vi "Create IRegisteredHandler.vi"(8 "error in (no error)":errorcluster, 11 "IWampMessage":refnum<class "IWampMessage.lvclass">) -> (0 "error out":errorcluster, 3 "IRegisteredHandler out":refnum<class "IRegisteredHandler.lvclass">)   [LabVIEW 2020, in "wamplv.lvlib"]
uses:
  wamplv.lvlib
  IRegisteredHandler.lvclass
  SerialisedMessages/IWampMessage/IWampMessage.lvclass
  RegisteredHandler JSON/RegisteredHandler JSON.lvclass
  C:/local/wamplv/Private/Requests/MessageReceivedHandlers/Registered/IRegisteredHandler.lvclass
  C:/local/wamplv/Private/Requests/MessageReceivedHandlers/IJsonMessageHandler/IJsonMessageHandler.lvclass
  SerialisedMessages/JSONMessage/JSONMessage.lvclass
  IJsonMessageHandler/IJsonMessageHandler.lvclass/IJsonMessageHandler.ctl
  RegisteredHandler MsgPack/RegisteredHandler MsgPack.lvclass
  C:/local/wamplv/Private/Requests/MessageReceivedHandlers/IMsgPackMessageHandler/IMsgPackMessageHandler.lvclass
  SerialisedMessages/MsgPackMessage/MsgPackMessage.lvclass
  IMsgPackMessageHandler/IMsgPackMessageHandler.lvclass/IMsgPackMessageHandler.ctl
  IJsonMessageHandler/IJsonMessageHandler.lvclass
  IMsgPackMessageHandler/IMsgPackMessageHandler.lvclass
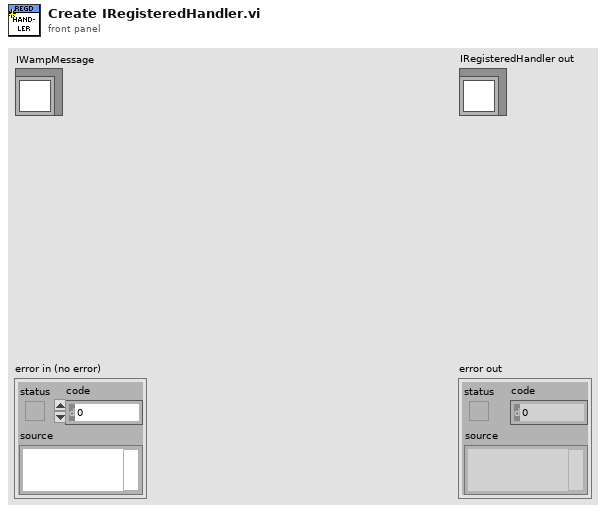
[diagram p1: front panel]
types:
  T1 = typedef "wamplv.lvlib/WAMP Client.lvclass/Serialisation.ctl" = enum16{"JSON", "MessagePack"}
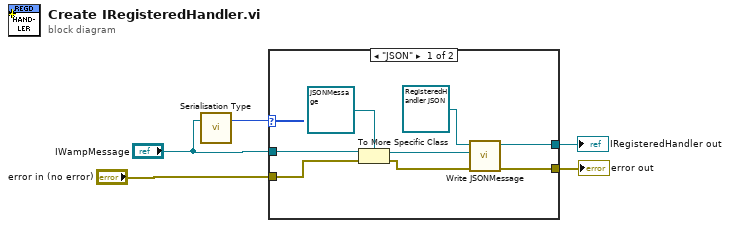
[diagram p0: block diagram]
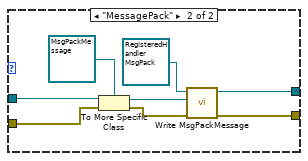
[diagram p2: hidden frame]
diagram:
  n1 = call-dynamic "Serialisation Type.vi"("IWampMessage in"="IWampMessage") -> ("Serialisation Type"=w5:T1)  [unwired: 2 in]
  n2 = case shown="\"JSON\"" w5 {
    tunnel: "IWampMessage" -> [w13 w21]
    tunnel: "error in (no error)" -> [w11 w20]
    tunnel: [w7 w15] -> w2
    tunnel: [w8 w16] -> w1
    frame "JSON" {
      n3 = To More Specific Class(target class=refnum<class "JSONMessage.lvclass"> refnum ("wamplv.lvlib:JSONMessage.lvclass"), reference=w13, error in=w11) -> (specific class reference=w10:refnum<class "JSONMessage.lvclass">, error out=w9:errorcluster)
      n4 = call "Write JSONMessage.vi"("error in (no error)"=w9, "wamplv.lvlib:JSONMessage.lvclass"=w10, "IJsonMessageHandler in"=refnum<class "RegisteredHandler JSON.lvclass"> refnum ("wamplv.lvlib:RegisteredHandler JSON.lvclass")) -> ("error out"=w8:errorcluster, "IJsonMessageHandler out"=w7:refnum<class "RegisteredHandler JSON.lvclass">)  [unwired: 7 in]
    }
    frame "MessagePack" {
      n5 = To More Specific Class(target class=refnum<class "MsgPackMessage.lvclass"> refnum ("wamplv.lvlib:MsgPackMessage.lvclass"), reference=w21, error in=w20) -> (specific class reference=w18:refnum<class "MsgPackMessage.lvclass">, error out=w17:errorcluster)
      n6 = call "Write MsgPackMessage.vi"("error in (no error)"=w17, "wamplv.lvlib:MsgPackMessage.lvclass"=w18, "IMsgPackMessageHandler in"=refnum<class "RegisteredHandler MsgPack.lvclass"> refnum ("wamplv.lvlib:RegisteredHandler MsgPack.lvclass")) -> ("error out"=w16:errorcluster, "IMsgPackMessageHandler out"=w15:refnum<class "RegisteredHandler MsgPack.lvclass">)  [unwired: 7 in]
    }
  }
  "error out" <- w1
  "IRegisteredHandler out" <- w2
